vi "Synchronize AWS S3 Content MAIN - App.vi"() -> ()   [LabVIEW 2026, in "Synchronize AWS S3 Content.lvlib" / "{TMPL} TLB`.lvclass"]
uses:
  {TMPL} TLB`.lvclass
  Application Components/Trigger API/System Trigger.ctl
  State Machine/State.ctl
  Core Components/Error Handler/TLB` Error Handler.lvclass
  Application Components/Configuration/{TMPL} Station Configuration.lvclass
  {TMPL} TLB`.lvclass/{TMPL} TLB`.ctl
  <vilib>/Utility/error.llb/Error Cluster From Error Code.vi
  <vilib>/ErrorRing/Error Ring.xnode
  Application Components/Trigger API/{TMPL} Trigger API.lvlib
  Synchronize AWS S3 Content.lvlib
  Core Components/Actions/Actions.lvlib
  Core Components/Dependencies/TLB`_Dependencies.lvlib
panel:
  out "error out":errorcluster
  out "State":string
  out "Status":string
  # "TLB` Template"
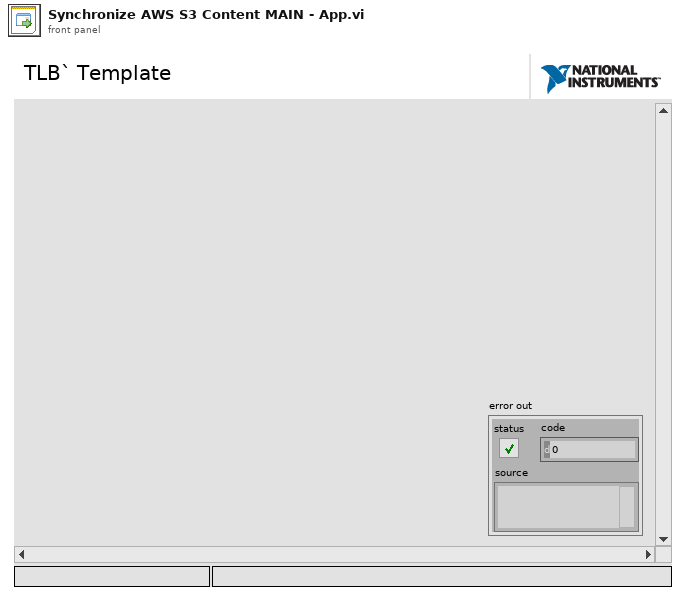
[diagram p1: front panel]
types:
  T1 = typedef "Synchronize AWS S3 Content.lvlib/{TMPL} TLB`.lvclass/State.ctl" = enum16{"<Startup>", "Idle", "<Shutdown>", "<Error>"}
  T2 = enum16{"Close Display", "Clear References", "Close Error Handler"}
  T3 = enum16{"Clear SR", "Set Display", "Set Shifter", "Initialize Events", "Init Q"}
  T4 = typedef "Synchronize AWS S3 Content.lvlib/{TMPL} Trigger API.lvlib/System Trigger.ctl" = enum16{"<None>", "Connect", "Start Acquisition", "Stop Acquisition", "Disconnect", "<Return to Safe State Actions>", "<Cache User Parameters>", "<Close Application>", "<Error>"}
  T5 = refnum<class "{TMPL} Station Configuration.lvclass">
  T6 = typedef "Synchronize AWS S3 Content.lvlib/_UI CORE Event References.ctl" = cluster{"Exit Event":refnum<user-event>, "State Indicator":refnum<user-event>, "Status Indicator":refnum<user-event>}
  T7 = typedef "Synchronize AWS S3 Content.lvlib/_UI APP Event References.ctl" = cluster{"Exit Event":refnum<user-event>}
  T8 = enum32{"Invalid", "Standard", "Closed", "Hidden", "Minimized", "Maximized"}
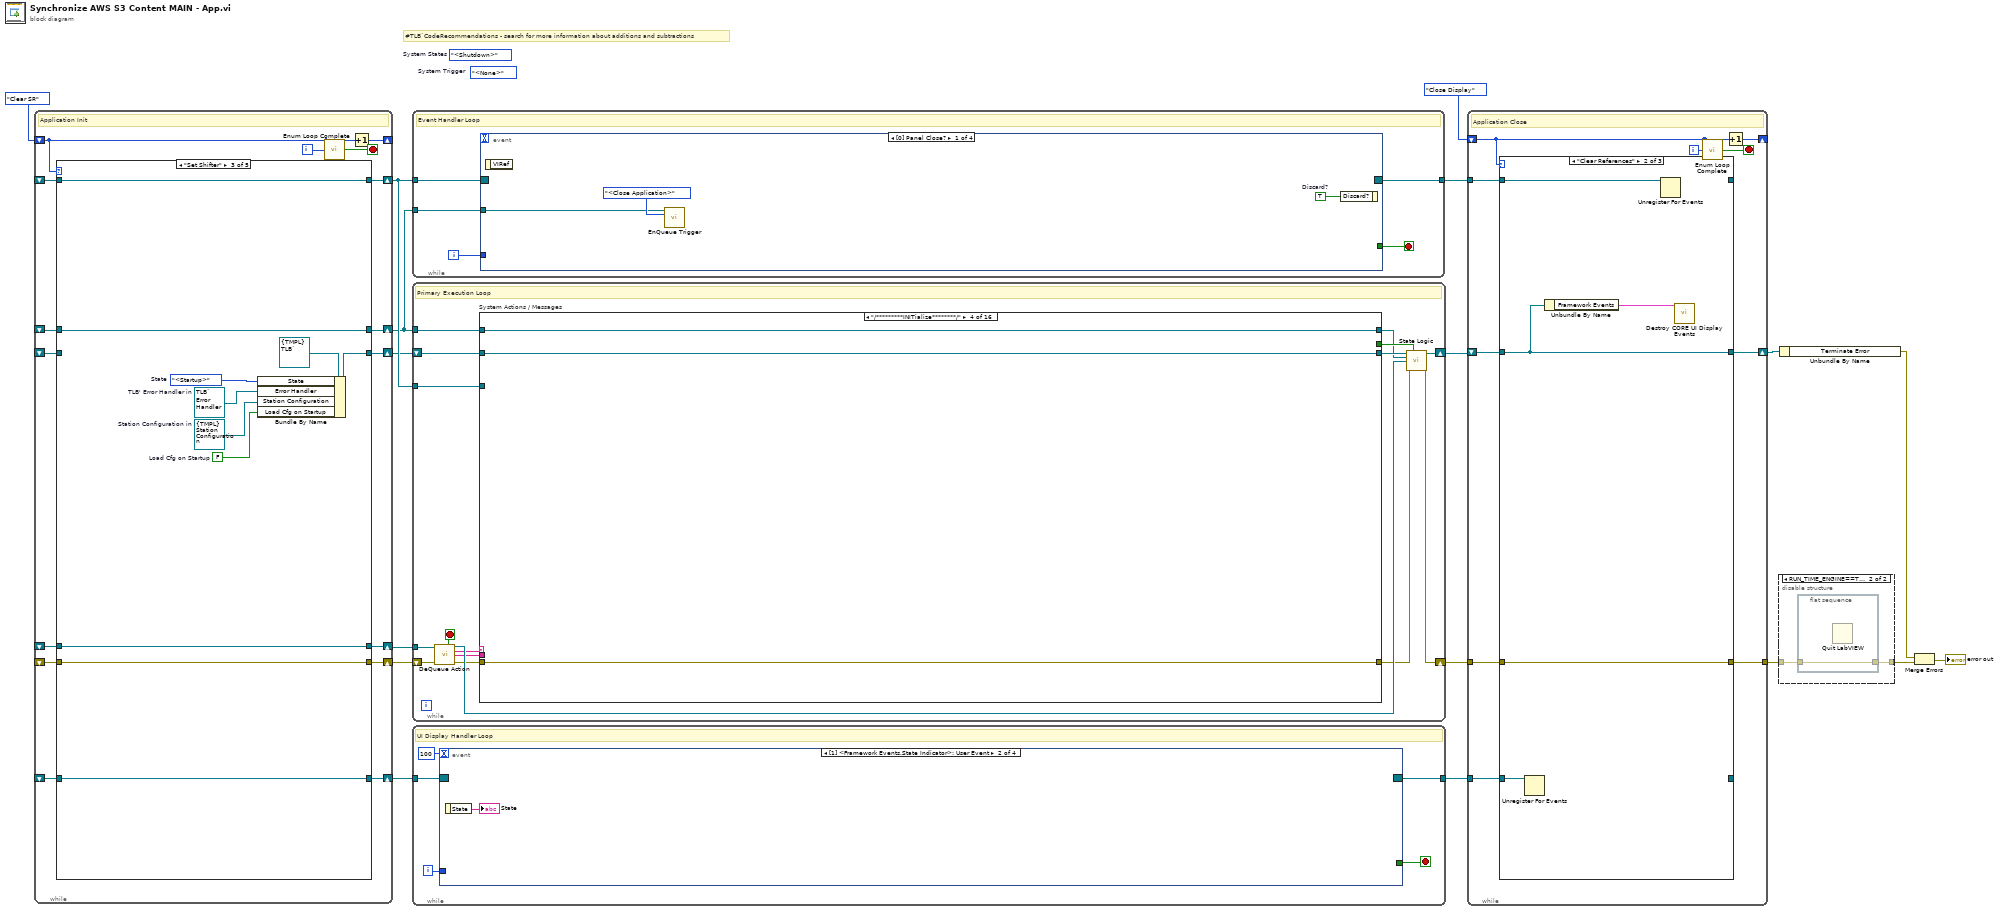
[diagram p0: block diagram]
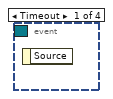
[diagram p2: hidden frame]
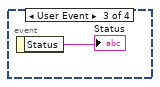
[diagram p3: hidden frame]
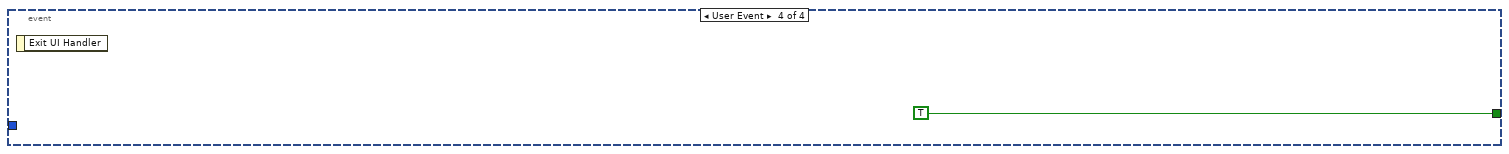
[diagram p4: hidden frame]
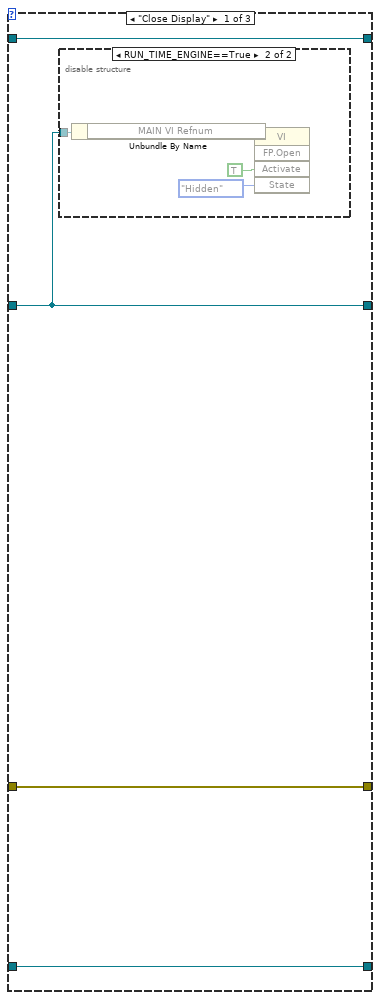
[diagram p6: hidden frame]
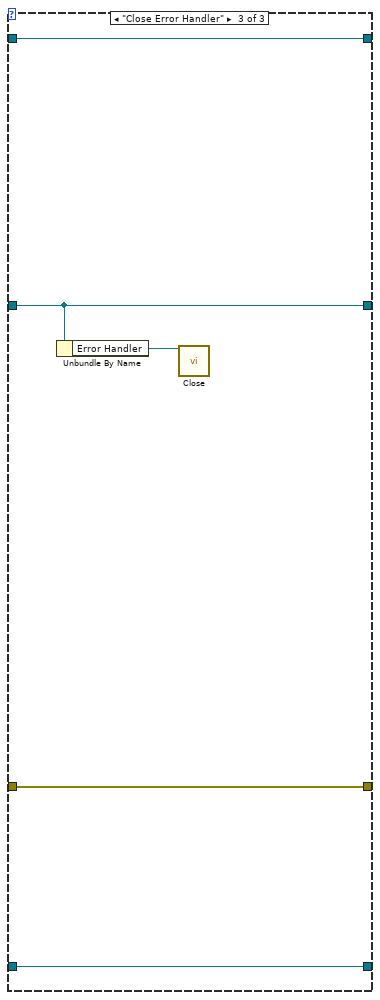
[diagram p8: hidden frame]
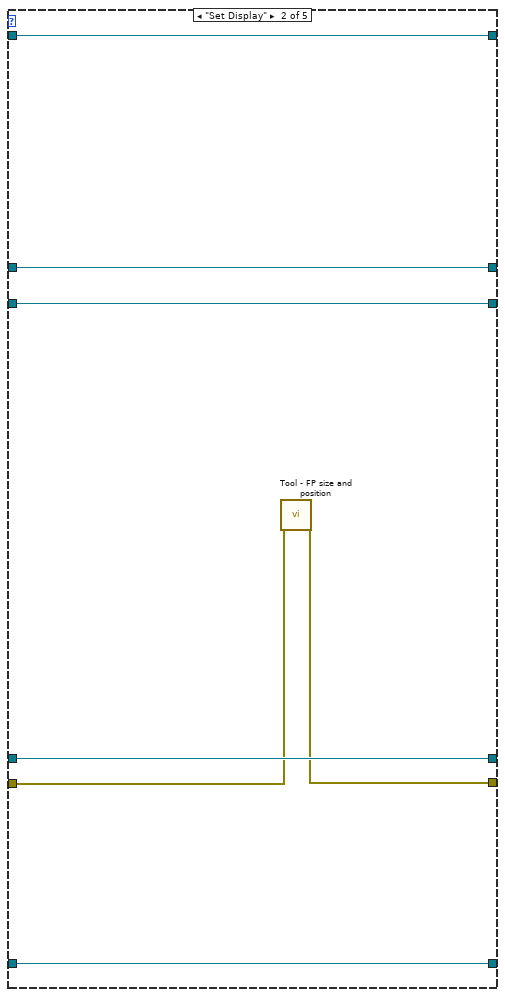
[diagram p10: hidden frame]
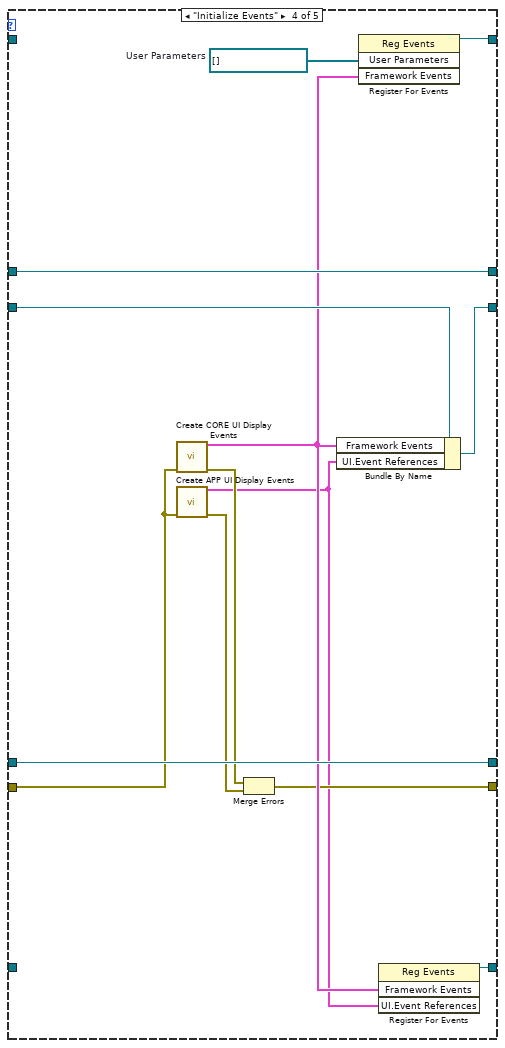
[diagram p11: hidden frame]
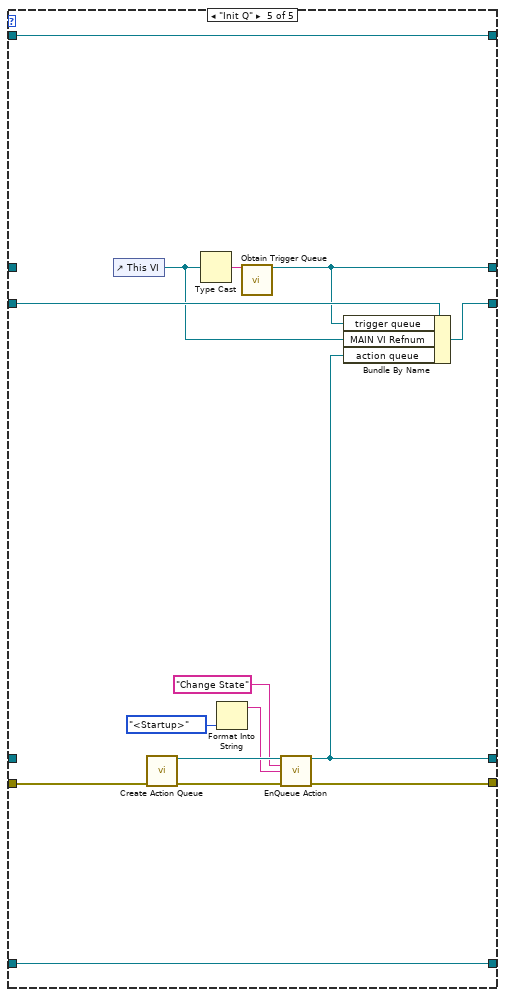
[diagram p12: hidden frame]
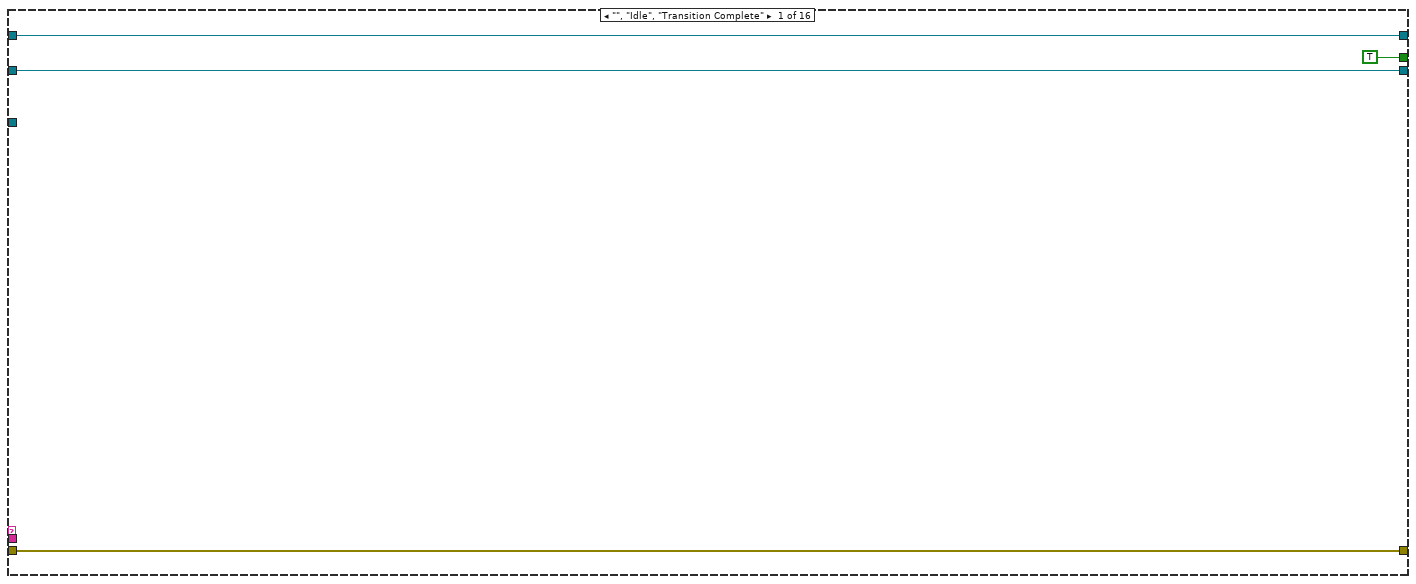
[diagram p13: hidden frame]
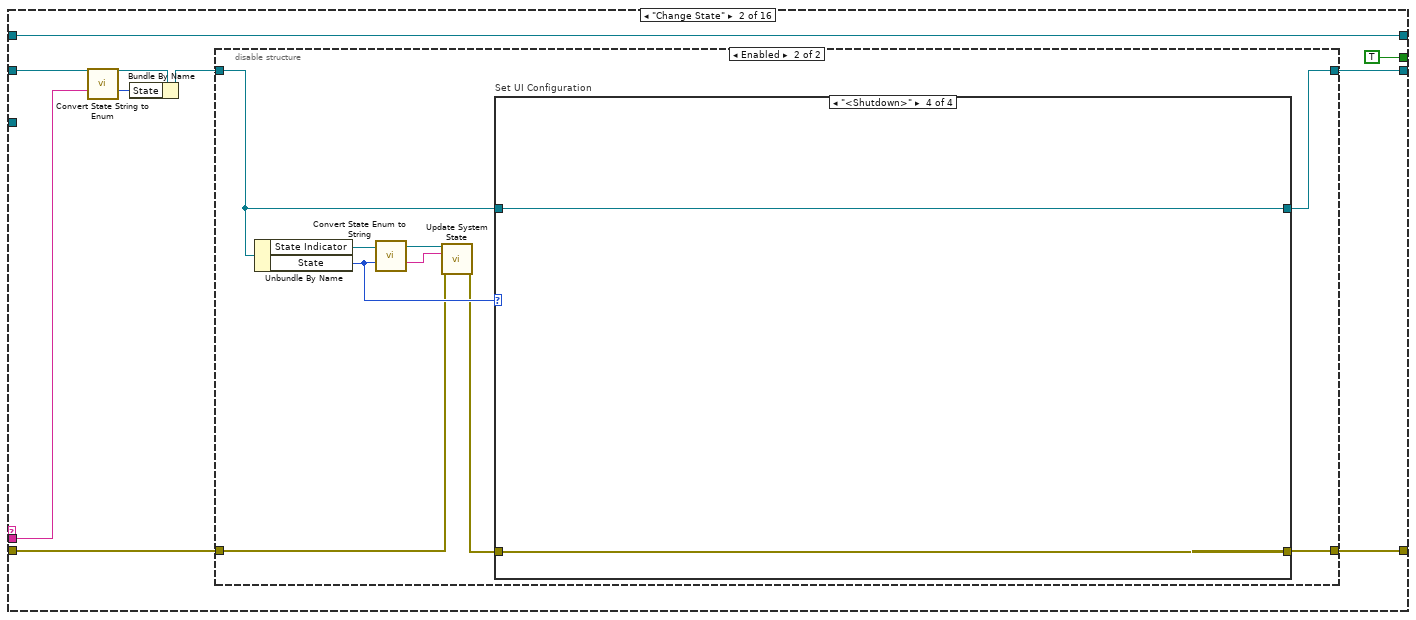
[diagram p14: hidden frame]
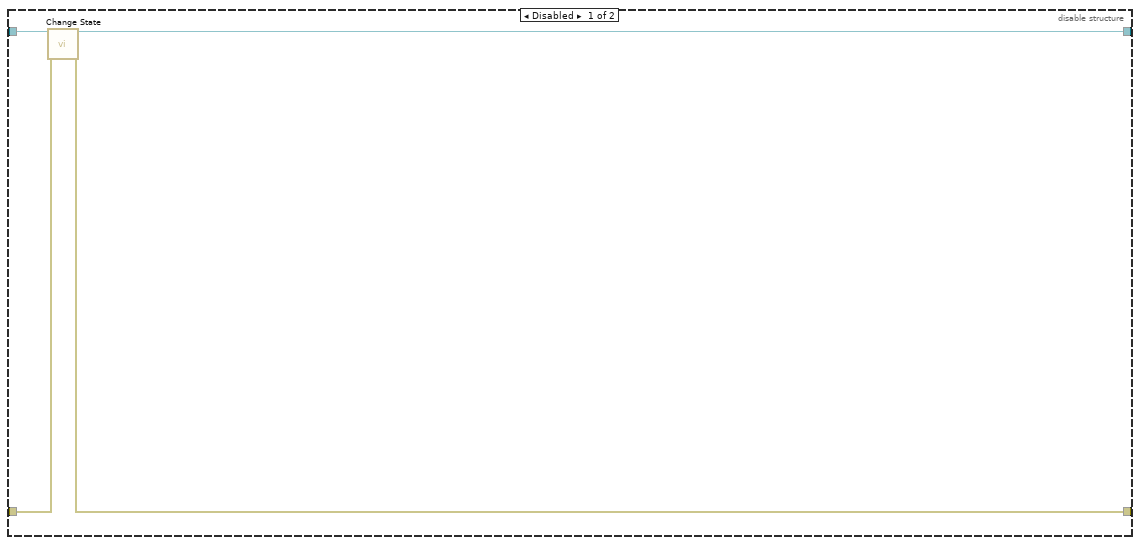
[diagram p15: hidden frame]
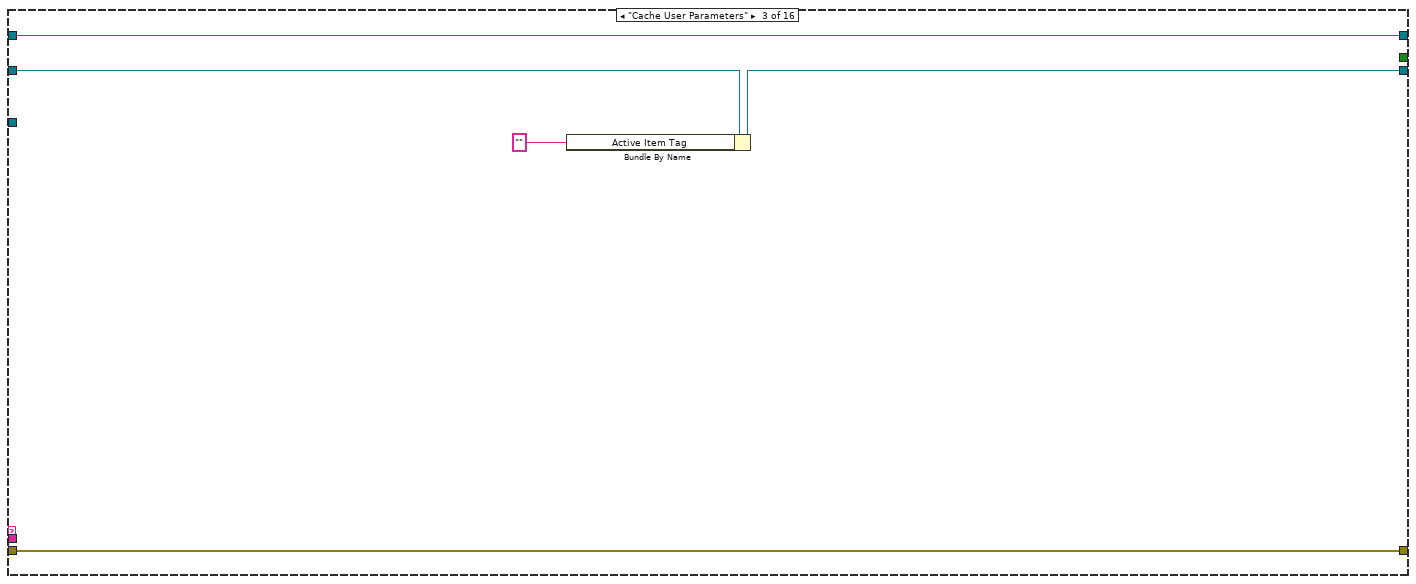
[diagram p19: hidden frame]
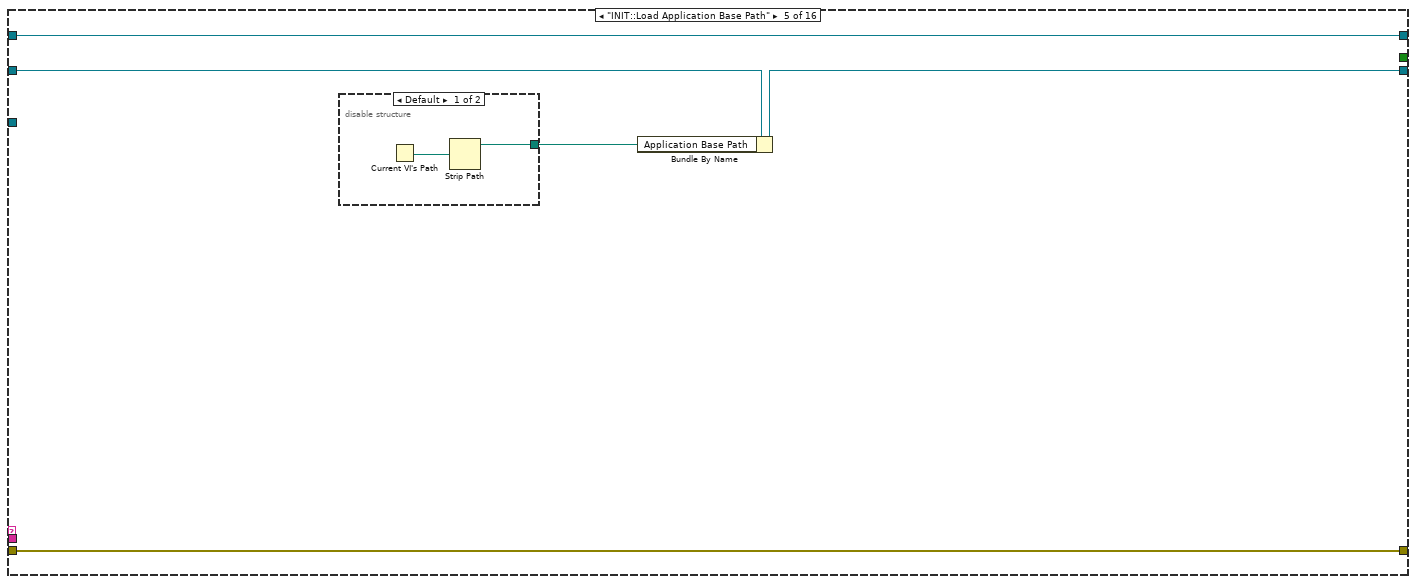
[diagram p20: hidden frame]
diagram:
  (unwired) State."<Shutdown>"  # System States
  (unwired) System_Trigger."<None>"  # System Trigger
  # "#TLB`CodeRecommendations - search for more information about additions and subtractions"
  n1 = while {
    shift-right: [w29] -> _
    shift-left: T3."Clear SR" -> [w18]
    shift-right: [w33] -> w17
    shift-left: _ -> [w28]
    shift-right: [w30] -> w12
    shift-left: _ -> [w27]
    shift-right: [w32] -> w11
    shift-left: _ -> [w26]
    shift-right: [w31] -> w10
    shift-left: _ -> [w25]
    shift-right: [w24] -> w6
    shift-left: _ -> [w23]
    shift-right: [w22] -> w9
    shift-left: _ -> [w21]
    i -> [w19]
    stop <- w20 stop-if-true
    # "Application Init"
    n2 = case shown="\"Set Shifter\"" w18 {
      tunnel: [_ w38 w51 w64 w65] -> w33
      tunnel: [_ w36 w50 w54 w71] -> w30
      tunnel: [_ w40 w46 w62 w77] -> w31
      tunnel: [_ w39 w49 w61 w79] -> w32
      tunnel: w28 -> [_ w38 w51 w64 _]
      tunnel: w27 -> [_ w37 w50 w53 w73]
      tunnel: w26 -> [_ w39 w49 _ w79]
      tunnel: w25 -> [_ w40 _ w63 w78]
      tunnel: [_ w35 w48 w60 w66] -> w24
      tunnel: w23 -> [_ w35 w48 w60 _]
      tunnel: [_ w34 w44 w58 w74] -> w22
      tunnel: w21 -> [_ w34 w44 _ w74]
      frame "Clear SR" {
      }
      frame "Set Display" {
        n3 = call "Tool - FP size and position.vi"("error in (no error)"=w37) -> ("error out"=w36:errorcluster)  [unwired: 17 in, 1 out]
      }
      frame "Set Shifter" {
        w41 = FALSE  # Load Cfg on Startup
        w42 = T5 refnum  # Station Configuration in
        w43 = refnum<class "TLB` Error Handler.lvclass"> refnum  # TLB' Error Handler in
        w47 = State."<Startup>"  # State
        n4 = Bundle By Name(cluster=refnum<class "{TMPL} TLB`.lvclass"> refnum ("TLB` Template.lvlib:TLB' Template.lvclass"), "State"=w47, "Error Handler"=w43, "Station Configuration"=w42, "Load Cfg on Startup"=w41) -> (w46:refnum<class "{TMPL} TLB`.lvclass">)
      }
      frame "Initialize Events" {
        w59 = refnum<vi>[] []  # User Parameters
        n5 = call "Create CORE UI Display Events.vi"("error in"=w53) -> ("Framework Events"=w57:T6, "error out"=w56:errorcluster)  [unwired: 13 in]
        n6 = call "Create APP UI Display Events.vi"("error in"=w53) -> ("UI.Event References"=w52:T7, "error out"=w55:errorcluster)  [unwired: 13 in]
        n7 = Merge Errors(w56, w55) -> (w54:errorcluster)
        n8 = Bundle By Name(cluster=w63, "Framework Events"=w57, "UI.Event References"=w52) -> (w62:refnum<class "{TMPL} TLB`.lvclass">)
        n9 = register-events(w59, w57) -> (reference out=w61:refnum<event-registration>)  [unwired: 2 in, 1 out]
        n10 = register-events(w57, w52) -> (reference out=w58:refnum<event-registration>)  [unwired: 2 in, 1 out]
      }
      frame "Init Q" {
        n11 = control-ref of="This VI"() -> (w76:refnum<vi>)
        n12 = call "Create Action Queue.vi"("error in"=w73) -> ("action queue out"=w70:refnum<queue>, "error out"=w72:errorcluster)  [unwired: 13 in]
        n13 = Type Cast(x=w76) -> (*(type *) &x=w67:string)  [unwired: 1 in]
        n14 = Format Into String(State."<Startup>" ("State")) -> (resulting string=w68:string)  [unwired: 3 in, 1 out]
        n15 = call "Obtain Trigger Queue.vi"("trigger queue name"=w67) -> ("trigger queue out"=w66:refnum<queue>)  [unwired: 13 in, 1 out]
        n16 = call "EnQueue Action.vi"("action queue in"=w70, "action"="Change State" ("Message Name"), "data in"=w68, "error in"=w72) -> ("action queue out"=w65:refnum<queue>, "error out"=w71:errorcluster)  [unwired: 10 in]
        n17 = Bundle By Name(cluster=w78, "trigger queue"=w66, "MAIN VI Refnum"=w76, "action queue"=w65) -> (w77:refnum<class "{TMPL} TLB`.lvclass">)
      }
    }
    n18 = call "Enum Loop Complete.vi"("Current State Enum"=w18, "Itteration"=w19) -> ("Loop Complete?"=w20:bool)  [unwired: 12 in, 1 out]
    n19 = Increment(x=w18) -> (x+1=w29:T3)
  }
  n20 = while {
    shift-right: [w90] -> w8
    shift-left: w12 -> [w85]
    shift-right: [w92] -> w13
    shift-left: w10 -> [w94]
    tunnel: w17 -> [w86]
    tunnel: w11 -> [w93]
    tunnel: w6 -> [w89]
    stop <- w84 stop-if-true
    # "Primary Execution Loop"
    n21 = call "DeQueue Action.vi"("action queue in"=w86, "error in"=w85) -> ("exit?"=w84:bool, "action queue out"=w95:refnum<queue>, "action"=w82:string, "action value"=w80:string, "error out"=w83:errorcluster)  [unwired: 8 in, 1 out]
    n22 = case "System Actions / Messages" shown="\"/*********INITialize********/\"" w82 {
      selector: w82 -> [_ _ _ _ _ _ _ _ _ _ _ _ _ _ _ w211]
      tunnel: [w99 w106 w132 w136 w137 w146 w155 w167 w174 w180 w183 w188 w193 w194 w206 w210] -> w87
      tunnel: w83 -> [w99 w105 w132 w136 w137 w149 w155 w167 w172 w180 w183 w187 w193 w195 w207 _]
      tunnel: w94 -> [w96 w104 w129 w135 w140 w147 w158 w166 w168 w179 w182 w190 w192 w198 w209 w213]
      tunnel: [w96 w100 w133 w135 w139 w152 w161 w166 w169 w179 w182 w190 w192 w197 w208 w213] -> w91
      tunnel: w93 -> [_ _ _ _ _ _ w159 _ _ _ _ _ _ _ _ _]
      tunnel: [w97 w107 w131 w134 w141 w153 w160 w165 w177 w178 w181 w185 w191 w201 w202 w212] -> w81
      tunnel: w89 -> [w97 w107 w131 w134 w141 w153 w160 w165 w177 w178 w181 w185 w191 w201 w202 w212]
      tunnel: [TRUE TRUE _ _ _ _ _ _ _ _ _ _ _ _ _ _] -> w88
      tunnel: w80 -> [_ w103 _ _ _ _ _ _ _ _ _ _ _ _ _ _]
      frame "", "Idle", "Transition Complete" {
      }
      frame "Change State" {
        n23 = call "Convert State String to Enum.vi"("state in"=w103) -> ("state out"=w102:T1)  [unwired: 13 in, 1 out]
        n24 = Bundle By Name(cluster=w104, "State"=w102) -> (w101:refnum<class "{TMPL} TLB`.lvclass">)
        n25 = disable-structure shown="Enabled" {
          disable-tunnel: [w112 w113] -> w106
          disable-tunnel: w105 -> [w111 w114]
          disable-tunnel: w101 -> [w110 w116]
          disable-tunnel: [w109 w115] -> w100
          frame Disabled {
            n26 = call "Change State.vi"("TLB' data in"=w110, "error in"=w111) -> ("TLB' data out"=w109:refnum<class "{TMPL} TLB`.lvclass">, "error out"=w112:errorcluster)  [unwired: 12 in]
          }
          frame Enabled {
            n27 = Unbundle By Name(w116) -> ("State Indicator"=w117:refnum<user-event>, "State"=w120:T1)
            n28 = call "Convert State Enum to String.vi"("state in"=w120) -> ("state out"=w118:string)  [unwired: 13 in, 1 out]
            n29 = call "Update System State.vi"("State Indicator"=w117, "system state message"=w118, "error in"=w114) -> ("error out"=w119:errorcluster)  [unwired: 12 in]
            n30 = case "Set UI Configuration" shown="\"<Shutdown>\"" w120 {
              tunnel: [w121 w124 w125 w128] -> w113
              tunnel: w119 -> [w121 w124 w125 w128]
              tunnel: [w122 w123 w126 w127] -> w115
              tunnel: w116 -> [w122 w123 w126 w127]
              frame "<Startup>" {
              }
              frame "Idle" {
              }
              frame "<Error>" {
              }
              frame "<Shutdown>" {
              }
            }
          }
        }
      }
      frame "Cache User Parameters" {
        n31 = Bundle By Name(cluster=w129, "Active Item Tag"="" ("User Data.Active Item Tag")) -> (w133:refnum<class "{TMPL} TLB`.lvclass">)
      }
      frame "/*********INITialize********/" {
      }
      frame "INIT::Load Application Base Path" {
        n32 = disable-structure shown="Default" {
          disable-tunnel: [w142 w144] -> w138
          frame condition #0 (active) {
            n33 = Current VI's Path() -> (path=w143:path)
            n34 = Strip Path(path=w143) -> (stripped path=w142:path)  [unwired: 1 out]
          }
          frame condition #1 {
            n35 = call <vilib>:"Application Directory.vi"() -> ("Application Directory"=w144:path)
          }
        }
        n36 = Bundle By Name(cluster=w140, "Application Base Path"=w138) -> (w139:refnum<class "{TMPL} TLB`.lvclass">)
      }
      frame "INIT::Initialize Error Handler" {
        n37 = Unbundle By Name(w147) -> ("Application Base Path"=w154:path)
        n38 = Unbundle By Name(w147) -> ("Error Handler"=w148:refnum<class "TLB` Error Handler.lvclass">)
        n39 = Build Path(base path=w154, name or relative path="System Level Errors\\System Errors.txt") -> (appended path=w150:path)
        n40 = call-dynamic "Open.vi"("error handler in"=w148, "error log path in"=w150, "error in"=w149) -> ("error handler out"=w151:refnum<class "TLB` Error Handler.lvclass">, "error out"=w146:errorcluster)  [unwired: 11 in]
        n41 = Bundle By Name(cluster=w147, "Error Handler"=w151) -> (w152:refnum<class "{TMPL} TLB`.lvclass">)
      }
      frame "INIT::Register User Parameters" {
        n42 = disable-structure shown="Enabled" {
          disable-tunnel: [w162 refnum<vi>[] [] ("User Parameter Controls")] -> w157
          frame Disabled {
            n43 = stacked-sequence "Stacked Sequence Structure :: Allows for a lot of controls" {
              tunnel: [w163] -> w162
              frame #0 {
                n44 = Build Array() -> (w163:void[])  [unwired: 4 in]
              }
            }
          }
          frame Enabled {
          }
        }
        n45 = Build Array (concatenate)(w157) -> (w156:refnum<vi>[])
        n46 = register-events(reference=w159, w156) -> ()  [unwired: 2 in, 2 out]
        n47 = Bundle By Name(cluster=w158, "User Parameter Controls"=w156) -> (w161:refnum<class "{TMPL} TLB`.lvclass">)
      }
      frame "INIT::FP Values" {
        # "#TLB`CodeRecommendations - initialize FP values here"
      }
      frame "CFG::Load Station Configuration" {
        n48 = Unbundle By Name(w168) -> ("Application Base Path"=w176:path)
        n49 = Unbundle By Name(w168) -> ("Station Configuration"=w171:T5)
        n50 = Build Path(base path=w176, name or relative path="System Configuration\\Station Configuration.ini") -> (appended path=w173:path)
        n51 = call-dynamic "Load Configuration.vi"("INI Station Configuration in"=w171, "INI file path in"=w173, "error in"=w172) -> ("INI Station Configuration out"=w170:T5, "error out"=w174:errorcluster)  [unwired: 11 in]
        n52 = Bundle By Name(cluster=w168, "Station Configuration"=w170) -> (w169:refnum<class "{TMPL} TLB`.lvclass">)
      }
      frame "/*********PRImary EXEcution********/" {
      }
      frame "/*********SHUTDOWN********/" {
      }
      frame "Exit" {
        w186 = refnum<class> refnum  # event data
        # "Don't wire 'Error In'\nMust Execute Regardless"
        n53 = Unbundle By Name(w190) -> ("Exit Event"=w184:refnum<user-event>)
        n54 = Generate User Event(user event=w184, event data cluster=w186) -> (error out=w189:errorcluster)  [unwired: 2 in, 1 out]
        n55 = Merge Errors(w187, w189) -> (w188:errorcluster)
      }
      frame "/*********ERRor Handler********/" {
      }
      frame "ERR::Log" {
        n56 = Unbundle By Name(w198) -> ("Error Handler"=w200:refnum<class "TLB` Error Handler.lvclass">)
        n57 = call-dynamic "Log.vi"("error handler in"=w200) -> ("error handler out"=w199:refnum<class "TLB` Error Handler.lvclass">, "error out"=w196:errorcluster)  [unwired: 13 in]
        n58 = Bundle By Name(cluster=w198, "Error Handler"=w199) -> (w197:refnum<class "{TMPL} TLB`.lvclass">)
        n59 = Merge Errors(w195, w196) -> (w194:errorcluster)
      }
      frame "ERR::Dialog" {
        n60 = Unbundle By Name(w209) -> ("Error Handler"=w205:refnum<class "TLB` Error Handler.lvclass">)
        n61 = call-dynamic "Dialog.vi"("error handler in"=w205, "trigger queue in"=w202) -> ("error handler out"=w204:refnum<class "TLB` Error Handler.lvclass">, "error out"=w203:errorcluster)  [unwired: 12 in]
        n62 = Merge Errors(w207, w203) -> (w206:errorcluster)
        n63 = Bundle By Name(cluster=w209, "Error Handler"=w204) -> (w208:refnum<class "{TMPL} TLB`.lvclass">)
      }
      frame Default {
        n64 = xnode "Error Ring"("parameter 0"=w211) -> ("error out"=w210:errorcluster)
      }
    }
    n65 = call "State Logic.vi"("TLB' data in"=w91, "process state logic enable"=w88, "trigger queue in"=w81, "action queue in"=w95, "error in"=w87) -> ("TLB' data out"=w92:refnum<class "{TMPL} TLB`.lvclass">, "error out"=w90:errorcluster)  [unwired: 9 in]
  }
  n66 = while {
    tunnel: w9 -> [w225]
    tunnel: [w221] -> w7
    i -> [w224]
    stop <- w223 stop-if-true
    # "UI Display Handler Loop"
    n67 = event shown="[1] <Framework Events.State Indicator>: User Event" {
      selector: w225 -> [_ _ _ _]
      dyn-events: [_ _ _ _] -> w221
      timeout: 100 -> [_ _ _ _]
      tunnel: w224 -> [_ _ _ _]
      tunnel: [_ _ _ TRUE] -> w223
      event Timeout {
        n68 = event-data() -> ()  [unwired: 2 out]
      }
      event User Event {
        n69 = event-data() -> ("State"=→"State":string)  [unwired: 1 out]
      }
      event User Event {
        n70 = event-data() -> ("Status"=→"Status":string)  [unwired: 1 out]
      }
      event User Event {
        n71 = event-data() -> ()  [unwired: 2 out]
      }
    }
  }
  n72 = while {
    tunnel: w11 -> [w232]
    tunnel: [w231] -> w14
    tunnel: w6 -> [w229]
    i -> [w230]
    stop <- w233 stop-if-true
    # "Event Handler Loop"
    n73 = event shown="[0] Panel Close?" {
      selector: w232 -> [_ _ _ _]
      dyn-events: [_ _ _ _] -> w231
      timeout: _ -> [_ _ _ _]
      tunnel: [_ _ TRUE ("NewVal") _] -> w233
      tunnel: w230 -> [_ _ _ _]
      tunnel: w229 -> [w234 _ w246 w250]
      event Panel Close? {
        w236 = TRUE  # Discard?
        n74 = event-data() -> ()  [unwired: 2 out]
        n75 = call "EnQueue Trigger.vi"("trigger queue in"=w234, "system trigger"=System_Trigger."<Close Application>" ("System Trigger")) -> ()  [unwired: 12 in, 2 out]
        n76 = event-data("Discard?"=w236) -> ()  [unwired: 1 in, 1 out]
      }
      event Mouse Down {
        n77 = event-data() -> ("Button"=w237:u16, "Mods.Double Click"=w238:bool)  [unwired: 1 out]
        n78 = Equal?(x=u16 2, y=w237) -> (x = y?=w240:bool)
        n79 = Compound Arithmetic op=AND(w240, w238) -> (w239:bool)
        n80 = case "Toggle Menu Visibility :: double RIGHT click on logo" shown="True" w239 {
          frame False {
          }
          frame True {
            n81 = property class="VI"() -> (reference out=w244:refnum<vi>, "TB.Visible"=w243:bool)  [unwired: 2 in, 1 out]
            n82 = Not(x=w243) -> (.not. x?=w242:bool)
            n83 = property class="VI"(reference=w244, "TB.Visible"=w242, "Front Panel.ShowMenuBar"=w242) -> ()  [unwired: 1 in, 2 out]
          }
        }
      }
      event User Event {
        n84 = event-data() -> ()  [unwired: 2 out]
        n85 = call "EnQueue Trigger.vi"("trigger queue in"=w246, "system trigger"=System_Trigger."<Close Application>" ("System Trigger")) -> ()  [unwired: 12 in, 2 out]
      }
      event Value Change {
        n86 = event-data() -> ()  [unwired: 2 out]
        n87 = call "EnQueue Trigger.vi"("trigger queue in"=w250, "system trigger"=System_Trigger."<Cache User Parameters>" ("System Trigger")) -> ("trigger queue out"=w249:refnum<queue>)  [unwired: 12 in, 1 out]
        n88 = event "use this event case to register a SPEICIFIC 'User Parameter' for a SPECIFIC action" shown="[0] Timeout" {
          selector: _ -> [_]
          dyn-events: _ -> [_]
          timeout: 0 -> [_]
          tunnel: w249 -> [_]
          event Timeout {
            n89 = event-data() -> ()  [unwired: 1 in, 1 out]
          }
        }
      }
    }
  }
  n90 = while {
    shift-right: [w261] -> _
    shift-left: T2."Close Display" -> [w254]
    tunnel: w14 -> [w259]
    tunnel: w8 -> [w260]
    tunnel: [w257] -> w16
    shift-right: [w256] -> w4
    shift-left: w13 -> [w258]
    tunnel: w7 -> [w255]
    i -> [w252]
    stop <- w253 stop-if-true
    # "Application Close"
    n91 = case shown="\"Clear References\"" w254 {
      tunnel: [w264 w274 w279] -> w257
      tunnel: [w263 w273 w276] -> w256
      tunnel: [w265 _ w278] -> _
      tunnel: w260 -> [w264 w274 w279]
      tunnel: w259 -> [w265 w272 w278]
      tunnel: w258 -> [w263 w273 w276]
      tunnel: w255 -> [w262 w270 w277]
      tunnel: [w262 _ w277] -> _
      frame "Close Display" {
        n92 = disable-structure shown="RUN_TIME_ENGINE==True" {
          disable-tunnel: w263 -> [_ w267]
          frame condition #0 (active) {
          }
          frame condition #1 {
            n93 = Unbundle By Name(w267) -> ("MAIN VI Refnum"=w266:refnum<vi>)
            n94 = invoke class="VI" method="FP.Open"(reference=w266, "Activate"=TRUE ("Activate?"), "State"=T8."Hidden") -> ()  [unwired: 2 in, 5 out]
          }
        }
      }
      frame "Clear References" {
        n95 = Unregister For Events(event registration refnum=w270) -> ()  [unwired: 1 in, 1 out]
        n96 = Unbundle By Name(w273) -> ("Framework Events"=w271:T6)
        n97 = Unregister For Events(event registration refnum=w272) -> ()  [unwired: 1 in, 1 out]
        n98 = call "Destroy CORE UI Display Events.vi"("UI display events in"=w271) -> ()  [unwired: 14 in, 1 out]
      }
      frame "Close Error Handler" {
        n99 = Unbundle By Name(w276) -> ("Error Handler"=w275:refnum<class "TLB` Error Handler.lvclass">)
        n100 = call-dynamic "Close.vi"("error handler in"=w275) -> ()  [unwired: 14 in, 1 out]
      }
    }
    n101 = call "Enum Loop Complete.vi"("Current State Enum"=w254, "Itteration"=w252) -> ("Loop Complete?"=w253:bool)  [unwired: 12 in, 1 out]
    n102 = Increment(x=w254) -> (x+1=w261:T2)
  }
  n103 = disable-structure shown="RUN_TIME_ENGINE==True" {
    disable-tunnel: [w280 w281] -> w2
    disable-tunnel: w16 -> [w280 w282]
    frame condition #0 (active) {
    }
    frame condition #1 {
      n104 = flat-sequence {
        tunnel: [w283] -> w281
        tunnel: w282 -> [w283]
        frame #0 {
          n105 = Quit LabVIEW() -> ()  [unwired: 1 in]
        }
      }
    }
  }
  n106 = Unbundle By Name(w4) -> ("Terminate Error"=w3:errorcluster)
  n107 = Merge Errors(w3, w2) -> (→"error out":errorcluster)
